vi "PH_PowerUnit_BaseClass.constructor.vi"(0 "name":string, 2 "data in":string, 5 "error in(no error)":errorcluster) -> (14 "i ref out":refnum<vi>, 16 "data out":string, 19 "error out":errorcluster)   [LabVIEW 2014, in "PH_PowerUnit_BaseClass.lvlib"]
doc: "This class is forseen to control a PreAmp Power Unit. Actually it controls several device layer classes. The head itself is fully operational, but should be used via the PHELIX_Sequencer class only. It has an own state machine.\n\nThis class is part of the PHELIX application layer.\n\nauthor: Stefan Götte, GSI\n\nLicense Agreement for this software:\n\nCopyright (C)\nGesellschaft für Schwerionenforschung, GSI\nPlanckstr. 1\n64291 Darmstadt\nGermany\n\nContact: D.Beck@gsi.de \n\nThis program is free software; you can redistribute it and/or modify it under the terms of the \nGNU General Public License as published by the Free Software Foundation; either version 2 of \nthe license, or (at your option) any later version.\n\nThis program is distributed in the hope that it will be useful, but WITHOUT ANY WARRANTY; \nwithout even the implied warranty of MERCHANTABILITY or FITNESS FOR A PARTICULAR PURPOSE. See the GNU General License for more details (http://www.gnu.org).\n\nGesellschaft für Schwerionenforschung, GSI\nPlanckstr. 1, 64291 Darmstadt, Germany\nFor all questions and ideas contact: M.Richter@gsi.de, H.Brand@gsi.de or D.Beck@gsi.de.\nLast update: 16-JUN-2004"
uses:
  PH_PowerUnit_BaseClass.lvlib
  PH_PSDBWriter/PH_PSDBWriter.lvlib
  PH_Class/PH_Class.lvlib
  CSCore/CSSystem/CSSystemLib/CSSystemLib.lvlib
  PH_SM_Class/PH_SM_Class.lvlib
  PH_StatusHandler/PH_StatusHandler.lvlib
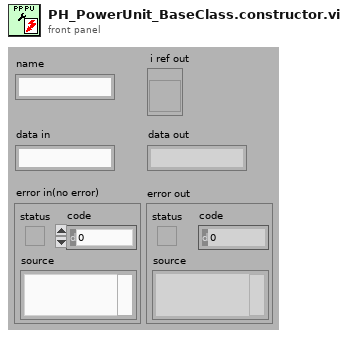
[diagram p1: front panel]
types:
  T1 = enum16{"SetAttribute", "GetAttribute", "CreateAttribute", "DestroyAttribute", "DestroyAllAtributes"}
  T2 = typedef "PH_PowerUnit_BaseClass.lvlib/PH_PowerUnit_BaseClass.i attribute.ctl" = cluster{"Constructor finished":bool, "PU":cluster{"In use":bool, "Service ID in use":i32, "GUI Ref":refnum<vi>}, "Enabling":cluster{"State":T3, "GUI Ref":refnum<vi>}, "Timing":cluster{"Last Shot":dbl, "Time between Shots [Sec]":dbl, "Waiting Time over?":bool, "Service ID Waiting Time":i32, "GUI Ref":refnum<vi>, "Instance":cluster{"Status":T4, "linked?":bool, "GUI Ref":refnum<vi>}}, "Sequencer":cluster{"SM State":string, "GUI Ref":refnum<vi>, "linked":bool}, "Subscribed Trendmssgs":cluster{"Tagname":string, "Status":T4, "linked?":bool, "Shot Condition":T4, "GUI Ref":refnum<vi>}[], "PP PU":T5, "Default Voltage (V)":dbl, "GUI Refs":T6, "PSDB data":cluster{"Shot Voltage [V]":dbl, "State TO SM":T7, "Write 2 early":bool}, "State TO SM":T7}
  T3 = typedef "PH_SystemInformation.lvlib/PH_SystemInformationEnabling State.ctl" = i32
  T4 = typedef "PH_StatusHandler.lvlib/PH_StatusHandler.Status.ctl" = i16
  T5 = typedef "PH_PP_Common.lvlib/PH_PP_Common.PUs.ctl" = enum16{"no Info", "PA-19mm-1", "PA-19mm-2", "PA-45mm-PILC", "PA-45mm-MAIN", "MA-PU-1", "MA-PU-2", "MA-PU-3", "MA-PU-4", "MA-PU-5", "MA-PU-6", "MA-FR", "MA-PILC", "PA-45mm-DP"}
  T6 = typedef "PH_PowerUnit_BaseClass.lvlib/PH_PowerUnit_BaseClass.GUI Refs.ctl" = cluster{"Delete Inst":refnum<vi>, "State TO SM":refnum<vi>, "State SM":refnum<vi>, "Fire":refnum<vi>}
  T7 = typedef "PH_PowerUnit_BaseClass.lvlib/PH_PowerUnit_BaseClass.SM States.ctl" = enum16{".", "Stand by", "Switch PU on", "Configure", "Set Default Voltage", "Set STANDBY", "Set READY", "Wait for Shot Cmd", "Open Dump Rods", "Open Ross Relais", "Close Ross Relais", "Switch PSU on", "Switch PSU off", "Charge", "Switch GD Channel on", "Close Dump Rods", "Rods-TO", "RR-TO", "PSU-TO", "Trigger-TO"}
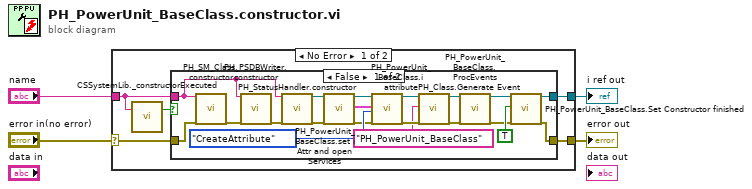
[diagram p0: block diagram]
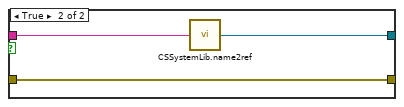
[diagram p2: hidden frame]
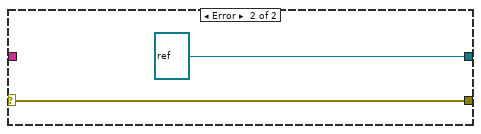
[diagram p3: hidden frame]
diagram:
  n1 = case shown="No Error" "error in(no error)" {
    selector: "error in(no error)" -> [w9 w34]
    tunnel: "name" -> [w6 _]
    tunnel: [w7 w34] -> w3
    tunnel: [w8 refnum<vi> refnum ("i ref out")] -> w2
    frame No Error {
      n2 = call "CSSystemLib._constructorExecuted.vi"("name"=w6) -> ("constructor executed?"=w5:bool)  [unwired: 18 in]
      n3 = case shown="False" w5 {
        tunnel: w9 -> [w14 w30]
        tunnel: [w21 w31] -> w8
        tunnel: [w18 w30] -> w7
        tunnel: w6 -> [w11 w32]
        frame False {
          n4 = call "PH_SM_Class.constructor.vi"("name"=w11, "error in"=w14) -> ("error out"=w13:errorcluster)  [unwired: 15 in, 2 out]
          n5 = call "PH_PSDBWriter.constructor.vi"("name"=w11, "error in"=w13) -> ("error out"=w19:errorcluster)  [unwired: 15 in, 2 out]
          n6 = call "PH_StatusHandler.constructor.vi"("name"=w11, "error in(no error)"=w19) -> ("i ref out"=w10:refnum<vi>, "error out"=w12:errorcluster)  [unwired: 15 in, 1 out]
          n7 = call "PH_PowerUnit_BaseClass.set i Attr and open Services.vi"("i ref in"=w10, "error in"=w12) -> ("i ref out"=w25:refnum<vi>, "i Attribhutes"=w27:T2, "error out"=w26:errorcluster)  [unwired: 15 in]
          n8 = call "PH_PowerUnit_BaseClass.i attribute.vi"("VI Refnum"=w25, "CLASS.i attribute"=w27, "Action"=T1."CreateAttribute", "error in (no error)"=w26) -> ("VI Refnum out"=w17:refnum<vi>, "error out"=w16:errorcluster)  [unwired: 13 in, 1 out]
          n9 = call "PH_Class.Generate Event.vi"("i ref in"=w17, "Class"="PH_PowerUnit_BaseClass", "error in (no error)"=w16) -> ("i ref out"=w23:refnum<vi>, "error out"=w24:errorcluster)  [unwired: 15 in]
          n10 = call "PH_PowerUnit_BaseClass.ProcEvents.vi"("i ref in"=w23, "error in (no error)"=w24) -> ("i ref out"=w22:refnum<vi>, "error out"=w20:errorcluster)  [unwired: 16 in]
          n11 = call "PH_PowerUnit_BaseClass.Set Constructor finished.vi"("VI in"=w22, "Constructor finished"=TRUE, "error in (no error)"=w20) -> ("VI out"=w21:refnum<vi>, "error out"=w18:errorcluster)  [unwired: 15 in]
        }
        frame True {
          n12 = call "CSSystemLib.name2ref.vi"("name"=w32) -> ("obj refnum"=w31:refnum<vi>)
        }
      }
    }
    frame Error {
    }
  }
  "i ref out" <- w2
  "error out" <- w3
